vi "ALTS-2015 Global Variables.vi"() -> ()   [LabVIEW 2013]
panel:
  in  "Error Log Updated?":bool
  in  "Exit Troubleshooter VI":bool
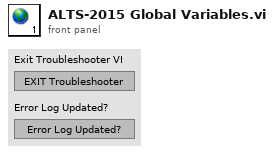
[diagram p1: front panel]
diagram:
